vi "Begin.vi"(8 "error in":errorcluster) -> (0 "error out":errorcluster)   [LabVIEW 2018]
doc: "Called before other user functions, this VI is expected to open initial I/O refnums, load in file data, and do all program initialization. Notice that the <B>error out</B> terminal is simply used for data flow. Wiring it to other structures or subVIs ensures that this VI runs first."
uses:
  <vilib>/Rock Robotics/WPI/DriverStation/WPI_DriverStationRobotMode2.ctl
  Typedefs/typedef_enum_Begin_State.ctl
  <vilib>/Rock Robotics/WPI/Joystick/WPI_JoystickDeviceEnum.ctl
  Typedefs/typedef_enum_refnums.ctl
  <vilib>/Rock Robotics/WPI/SafetyOutput/WPI_SafetyOutputConfigMenu.ctl
  <vilib>/Rock Robotics/SystemInterfaces/DIO/FPGA_DIOChannel.ctl
  <vilib>/Rock Robotics/SystemInterfaces/DIO/FPGA_DIOPWMChannel.ctl
  <vilib>/Rock Robotics/WPI/Solenoid/WPI_SolenoidChannel.ctl
  <vilib>/Rock Robotics/WPI/ThirdParty/Phoenix-LabVIEW/Motor Controller/Controls/CTRE_Phoenix_MotorControl_FeedbackDevice.ctl
  Robot Global Data.vi
  <vilib>/Rock Robotics/Network Tables/NT Write Number.vi
  <vilib>/Rock Robotics/WPI/Counter/WPI_CounterDigitalInputToDigitalSource.vi
  <vilib>/Rock Robotics/WPI/RobotDrive/WPI_RobotDriveOpen4MotorWithSPARK.vi
  <vilib>/Rock Robotics/WPI/MotorControl/WPI_MotorControlOpen SPARK.vi
  <vilib>/Rock Robotics/WPI/Switch/WPI_SwitchOpenLimit.vi
  <vilib>/Rock Robotics/WPI/Solenoid/WPI_SolenoidOpenDouble.vi
  <vilib>/Rock Robotics/WPI/Utilities/WPI_GetSetVariantRefNum.vi
  <vilib>/Rock Robotics/Network Tables/NT Write String Array.vi
  <vilib>/Rock Robotics/WPI/Gyro/WPI_GyroXRS450_SPI_Open.vi
  <vilib>/Rock Robotics/SystemInterfaces/spilib/spi_bus.ctl
  <vilib>/Rock Robotics/SystemInterfaces/AI/FPGA_AIChannel.ctl
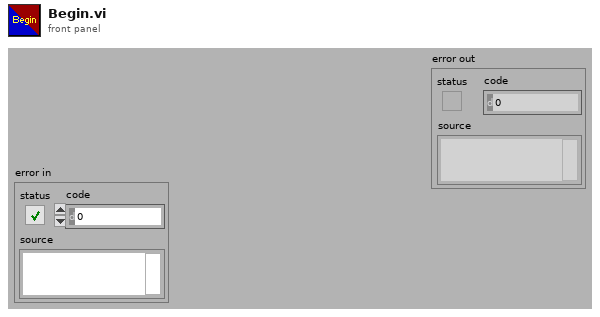
[diagram p1: front panel]
types:
  T1 = typedef "typedef_enum_Begin_State.ctl" = enum16{"Network_Setup", "Joy_Stick_Setup", "Drive_Train_Setup", "Ball_Intake_Setup", "Wrist_Setup", "Hatch_Deploy_Setup", "Compressor_Setup", "Lift_Setup", "Gyro_Setup", "Stop"}
  T2 = typedef "WPI_DriverStationRobotMode2.ctl" = enum16{"Autonomous Disabled", "Autonomous Enabled", "Teleop Disabled", "Teleop Enabled", "Disconnected", "Finish", "Test Disabled", "Test Enabled", "Emergency Stopped"}
  T3 = typedef "typedef_enum_refnums.ctl" = enum16{"Joy_L", "Joy_R", "Drive_Motors", "Intake_Motor", "Wrist_Solenoid", "Hatch_Solenoid", "Compressor", "Lift_Motor", "Lift_Motor_2", "Gyro", "Drive_Enc_L", "Drive_Enc_R", "Lift_Lower_Limit", "Lift_Upper_Limit", "Ball_Switch", "Jump_Solenoid"}
  T4 = typedef "WPI_JoystickDeviceEnum.ctl" = enum16{"USB 0", "USB 1", "USB 2", "USB 3", "USB 4", "USB 5"}
  T5 = typedef "WPI_SafetyOutputConfigMenu.ctl" = enum16{"Enable", "Disable"}
  T6 = typedef "FPGA_DIOPWMChannel.ctl" = enum8{"PWM 0", "PWM 1", "PWM 2", "PWM 3", "PWM 4", "PWM 5", "PWM 6", "PWM 7", "PWM 8", "PWM 9", "PWM MXP 0", "PWM MXP 1", "PWM MXP 2", "PWM MXP 3", "PWM MXP 4", "PWM MXP 5", "PWM MXP 6", "PWM MXP 7", "PWM MXP 8", "PWM MXP 9", "Invalid"}
  T7 = typedef "WPI_SolenoidChannel.ctl" = enum8{"Solenoid 0", "Solenoid 1", "Solenoid 2", "Solenoid 3", "Solenoid 4", "Solenoid 5", "Solenoid 6", "Solenoid 7", "Invalid"}
  T8 = typedef "FPGA_DIOChannel.ctl" = enum8{"DIO 0", "DIO 1", "DIO 2", "DIO 3", "DIO 4", "DIO 5", "DIO 6", "DIO 7", "DIO 8", "DIO 9", "DIO MXP 0", "DIO MXP 1", "DIO MXP 2", "DIO MXP 3", "DIO MXP 4", "DIO MXP 5", "DIO MXP 6", "DIO MXP 7", "DIO MXP 8", "DIO MXP 9", "DIO MXP 10", "DIO MXP 11", "DIO MXP 12", "DIO MXP 13", "DIO MXP 14", "DIO MXP 15", "SPI Port CS1", "SPI Port CS2", "SPI Port CS3", "SPI Port MISO", "SPI Port MOSI", "Invalid"}
  T9 = enum16{"FollowerType_PercentOutput", "FollowerType_AuxOutput1"}
  T10 = typedef "spi_bus.ctl" = enum16{"SPI On-Board, CS0", "SPI On-Board, CS1", "SPI On-Board, CS2", "SPI On-Board, CS3", "SPI MXP", "Invalid"}
  T11 = typedef "typedef_enum_refnums.ctl" = enum16{"Joy_L", "Joy_R", "Drive_Motors", "Intake_Motor", "Wrist_Solenoid", "Hatch_Solenoid", "Compressor", "Lift_Motor", "Lift_Motor_2", "Gyro", "Potentio", "Drive_Enc_L", "Drive_Enc_R", "Lift_Lower_Limit", "Lift_Upper_Limit", "Ball_Switch", "Jump_Solenoid"}
  T12 = typedef "FPGA_AIChannel.ctl" = enum8{"AI 0", "AI 1", "AI 2", "AI 3", "AI MXP 0", "AI MXP 1", "AI MXP 2", "AI MXP 3", "Invalid"}
  T13 = typedef "WPI_JoystickDevRef.ctl" = cluster{"Device":T4}
  T14 = typedef "WPI_RobotDriveDevRef.ctl" = cluster{"DevStatus":errorcluster, "Motors[]":T15[], "Square Inputs":bool, "Max Output":dbl}
  T15 = typedef "WPI_MotorControlDeviceRef.ctl" = cluster{"DeviceStatus":errorcluster, "Type":T16, "PWM":cluster{"PWM Channel":T6, "DeadBand":T17}, "CAN":cluster{"Device Number":u8, "SetOutput VI Ref":variant, "GetOutput VI Ref":variant, "Enable VI Ref":variant, "Disable VI Ref":variant, "Data":variant}, "Invert":bool, "DIO PWM":cluster{"PWM \"Enable\" Channel":T6, "DIOChannel":T8, "PWM Rate":dbl}}
  T16 = typedef "WPI_MotorControlType.ctl" = enum16{"PWM", "CAN", "DIO PWM"}
  T17 = typedef "WPI_PWMDeadband.ctl" = cluster{"Name":string, "maxPositivePwm":i32, "minPositivePwm":i32, "centerPwm":i32, "maxNegativePwm":i32, "minNegativePwm":i32, "angularRange":u16}
  T18 = typedef "WPI_DigitalInputDevRef.ctl" = cluster{"DevStatus":errorcluster, "DIO Channel":T8}
  T19 = typedef "FPGA_CounterEncoderSourceConvertionLVSourceType.ctl" = cluster{"DevStatus":errorcluster, "AnalogTriggerMode?":bool, "DigitalMode":cluster{"DIO Channel":T20}, "AnalogTriggerMode":cluster{"AnalogTriggerIndex":T21, "OutputType":T22}}
  T20 = typedef "FPGA_DIODigitalSourceChannel.ctl" = enum8{"DIO 0", "DIO 1", "DIO 2", "DIO 3", "DIO 4", "DIO 5", "DIO 6", "DIO 7", "DIO 8", "DIO 9", "DIO MXP 0", "DIO MXP 1", "DIO MXP 2", "DIO MXP 3", "DIO MXP 4", "DIO MXP 5", "DIO MXP 6", "DIO MXP 7", "DIO MXP 8", "DIO MXP 9", "DIO MXP 10", "DIO MXP 11", "DIO MXP 12", "DIO MXP 13", "DIO MXP 14", "DIO MXP 15", "SPI Port CS1", "SPI Port CS2", "SPI Port CS3", "SPI Port MISO", "SPI Port MOSI", "Disabled"}
  T21 = typedef "FPGA_AnalogTriggerIndex.ctl" = enum8{"Trig 0", "Trig 1", "Trig 2", "Trig 3", "Trig 4", "Trig 5", "Trig 6", "Trig 7", "Invalid"}
  T22 = typedef "FPGA_AnalogTriggerOutType.ctl" = enum16{"InWindow", "TriggerState", "Rising", "Falling"}
  T23 = typedef "WPI_EncoderDevRef.ctl" = cluster{"DevStatus":errorcluster, "EncoderIndex":T24, "CounterIndex":T25, "DistancePerCount":dbl, "Decoding Type":T26}
  T24 = typedef "FPGA_EncoderIdx.ctl" = enum8{"Enc 0", "Enc 1", "Enc 2", "Enc 3", "Enc 4", "Enc 5", "Enc 6", "Enc 7", "Invalid"}
  T25 = typedef "FPGA_CounterCtrSystemIndex.ctl" = enum8{"Ctr 0", "Ctr 1", "Ctr 2", "Ctr 3", "Ctr 4", "Ctr 5", "Ctr 6", "Ctr 7", "Invalid"}
  T26 = typedef "WPI_EncoderType.ctl" = enum16{"1x", "2x", "4x"}
  T27 = typedef "WPI_SwitchDevRef.ctl" = cluster{"DevStatus":errorcluster, "DIO Channel":T8, "CntIndex":T25, "Normally Closed":bool}
  T28 = typedef "WPI_SolenoidDevRef.ctl" = cluster{"DevStatus":errorcluster, "Pneumatics Control Module":u8, "Forward Solenoid Channel":T7, "Reverse Solenoid Channel":T7}
  T29 = typedef "WPI_CompressorDevRef.ctl" = cluster{"DevStatus":errorcluster, "Pneumatics Control Module":u8}
  T30 = typedef "CTRE_Phoenix_MotorControl_FeedbackDevice.ctl" = i8
  T31 = typedef "WPI_GyroDevRef.ctl" = cluster{"DevStatus":errorcluster, "Analog Channel":T12, "Gain (VoltsPerDegree/Second)":dbl, "Gyro Type":enum16{"Analog", "XRS450"}, "Handle":i32, "SPI Bus":T10, "Device Found":bool, "Sample Rate":dbl, "Calibrate On Open":bool, "Offset":dbl}
  T32 = typedef "WPI_PotentiometerDevRef.ctl" = cluster{"DevStatus":errorcluster, "Analog Channel":T12, "Invert Output":bool}
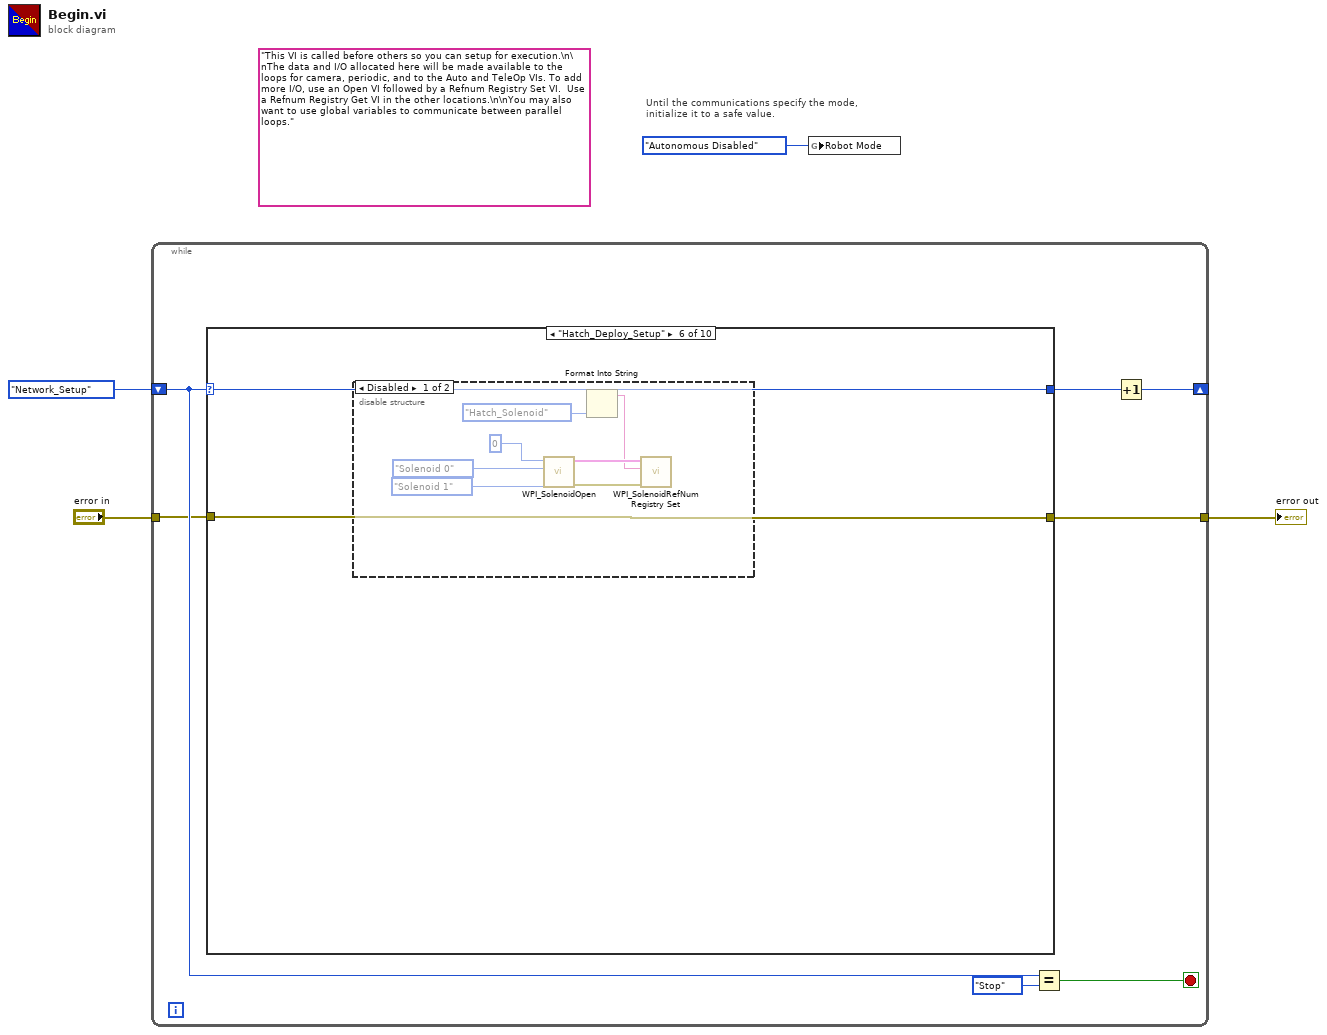
[diagram p0: block diagram]
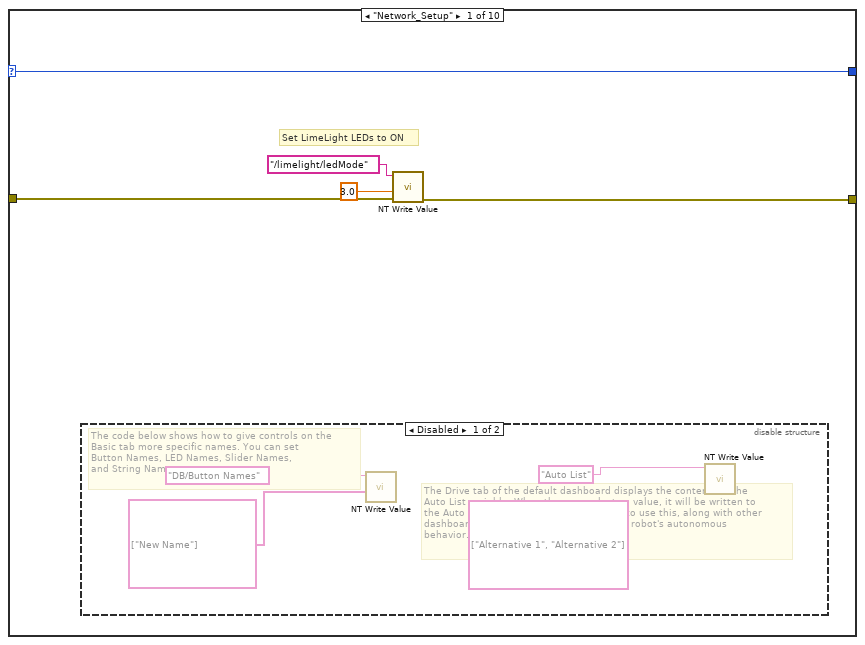
[diagram p2: hidden frame]
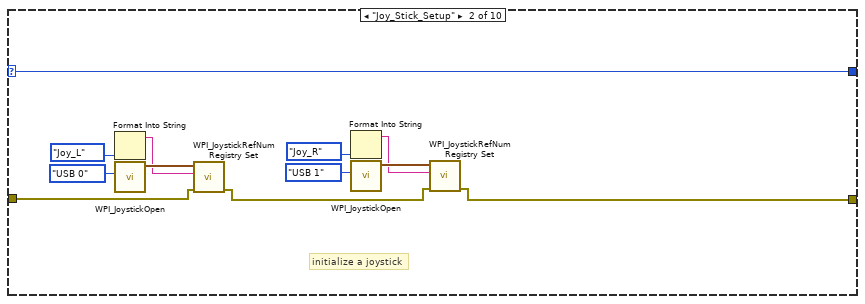
[diagram p4: hidden frame]
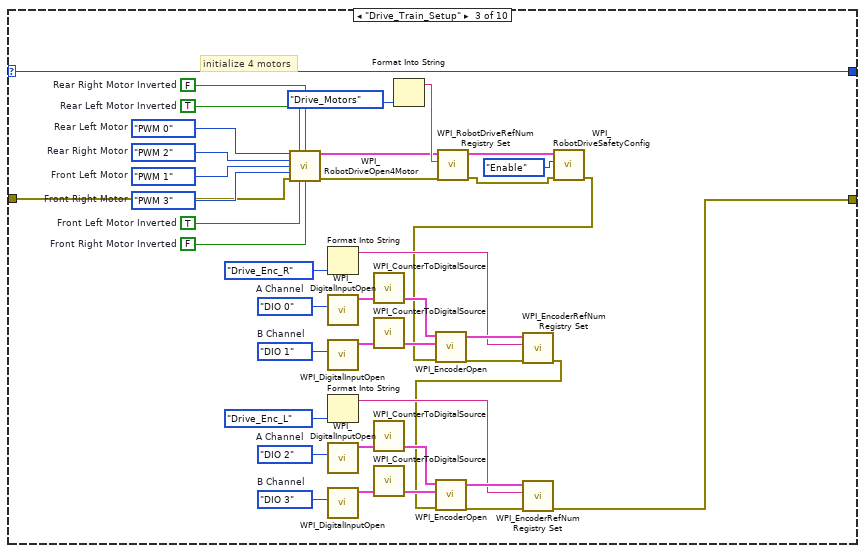
[diagram p5: hidden frame]
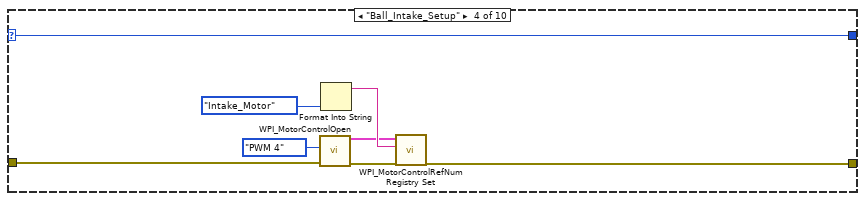
[diagram p6: hidden frame]
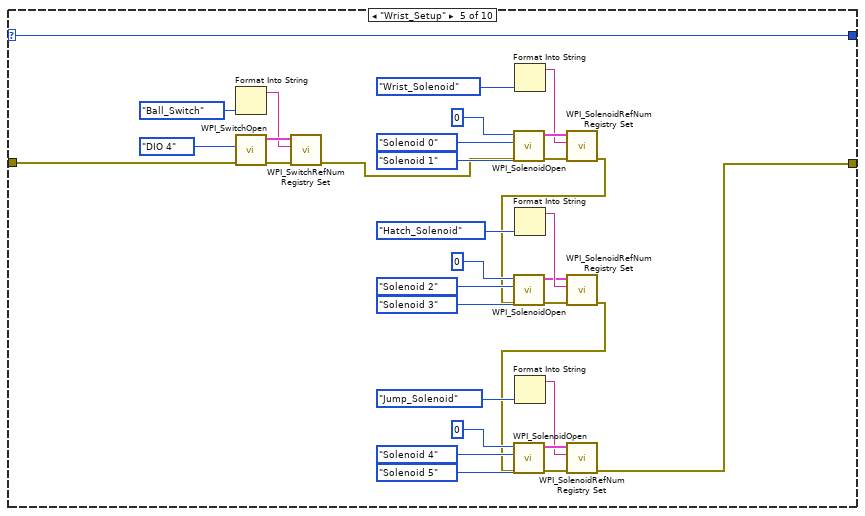
[diagram p7: hidden frame]
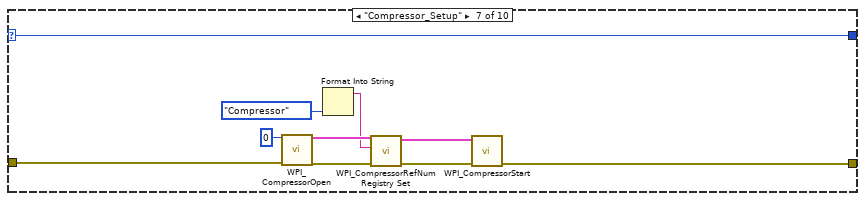
[diagram p9: hidden frame]
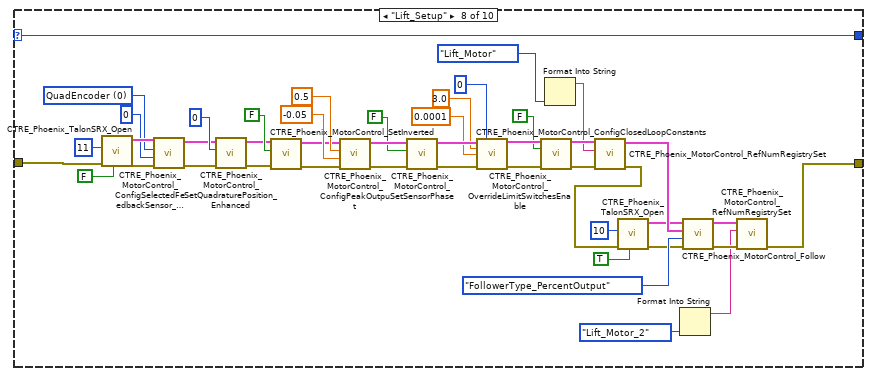
[diagram p10: hidden frame]
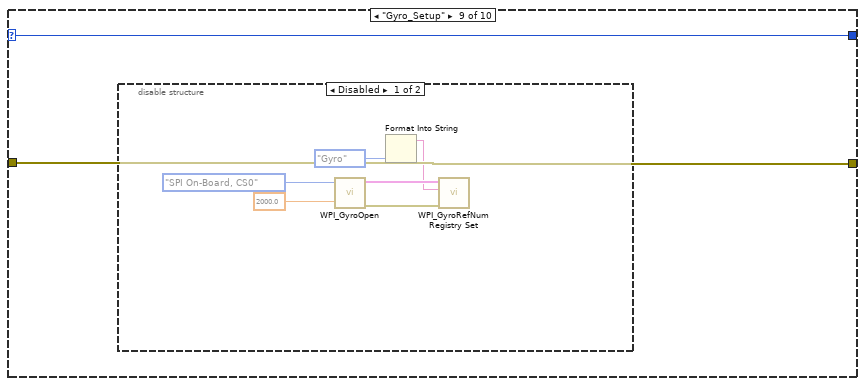
[diagram p11: hidden frame]
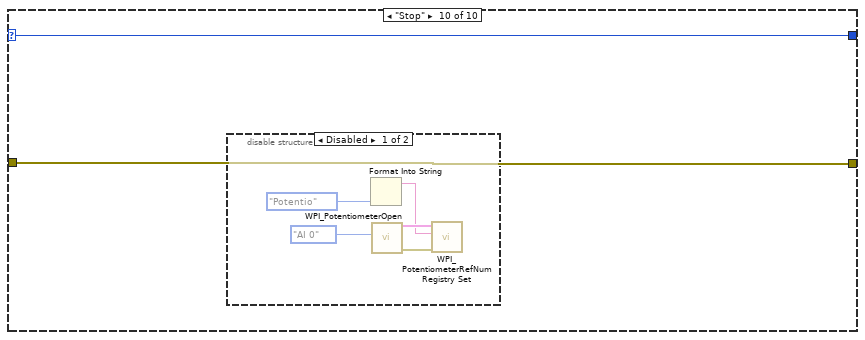
[diagram p13: hidden frame]
diagram:
  (unwired) "This VI is called before others so you can setup for execution.\n\nThe data and I/O allocated here will be made available to the loops for camera, periodic, and to the Auto and TeleOp VIs. To add more I/O, use an Open VI followed by a Refnum Registry Set VI.  Use a Refnum Registry Get VI in the other locations.\n\nYou may also want to use global variables to communicate between parallel loops."
  # "Until the communications specify the mode,\ninitialize it to a safe value."
  n1 = while {
    shift-right: [w10] -> _
    shift-left: typedef_enum_Begin_State."Network_Setup" ("Enum") -> [w8]
    tunnel: "error in" -> [w6]
    tunnel: [w5] -> w1
    stop <- w9 stop-if-true
    n2 = case shown="\"Hatch_Deploy_Setup\"" w8 {
      selector: w8 -> [w16 w32 w72 w80 w112 w114 w131 w176 w178 w186]
      tunnel: [w16 w32 w72 w80 w112 w114 w131 w176 w178 w186] -> w11
      tunnel: w6 -> [w13 w23 w38 w74 w85 w113 w123 w140 w177 w185]
      tunnel: [w12 w22 w33 w73 w81 w113 w122 w132 w177 w185] -> w5
      frame "Network_Setup" {
        # "Set LimeLight LEDs to ON"
        n3 = disable-structure shown="Disabled" {
          frame Disabled {
            # "The Drive tab of the default dashboard displays the contents of the\nAuto List variable. When the user selects a value, it will be written to\nthe Auto Selector variable. You may want to use this, along with other\ndashboard inputs, to let drivers define the robot's autonomous\nbehavior."
            # "The code below shows how to give controls on the\nBasic tab more specific names. You can set\nButton Names, LED Names, Slider Names,\nand String Names."
            n4 = call-poly <vilib>:"NT Write Value.vi"("String Array"=string[] ["New Name"], "Name"="DB/Button Names") -> ()  [unwired: 9 in, 1 out]
            n5 = call-poly <vilib>:"NT Write Value.vi"("String Array"=string[] ["Alternative 1", "Alternative 2"], "Name"="Auto List") -> ()  [unwired: 9 in, 1 out]
          }
          frame Enabled {
          }
        }
        n6 = call-poly <vilib>:"NT Write Value.vi"("error in"=w13, "Numeric"=3.0, "Name"="/limelight/ledMode") -> ("error out"=w12:errorcluster)  [unwired: 8 in]
      }
      frame "Joy_Stick_Setup" {
        # "initialize a joystick"
        n7 = Format Into String(typedef_enum_refnums."Joy_L" ("Enum")) -> (resulting string=w26:string)  [unwired: 3 in, 1 out]
        n8 = call <vilib>:"WPI_JoystickOpen.vi"("JoystickDevice"=WPI_JoystickDeviceEnum."USB 0") -> ("JoystickDevRef"=w28:T13)  [unwired: 10 in]
        n9 = call <vilib>:"WPI_JoystickRefNum Registry Set.vi"("error in (no error)"=w23, "refnum name"=w26, "JoystickDevRef"=w28) -> ("error out"=w21:errorcluster)  [unwired: 7 in, 1 out]
        n10 = Format Into String(typedef_enum_refnums."Joy_R" ("Enum")) -> (resulting string=w24:string)  [unwired: 3 in, 1 out]
        n11 = call <vilib>:"WPI_JoystickOpen.vi"("JoystickDevice"=WPI_JoystickDeviceEnum."USB 1") -> ("JoystickDevRef"=w31:T13)  [unwired: 10 in]
        n12 = call <vilib>:"WPI_JoystickRefNum Registry Set.vi"("error in (no error)"=w21, "refnum name"=w24, "JoystickDevRef"=w31) -> ("error out"=w22:errorcluster)  [unwired: 7 in, 1 out]
      }
      frame "Drive_Train_Setup" {
        w39 = FALSE  # Rear Right Motor Inverted
        w40 = TRUE  # Front Left Motor Inverted
        w41 = FALSE  # Front Right Motor Inverted
        w42 = TRUE  # Rear Left Motor Inverted
        w43 = FPGA_DIOPWMChannel."PWM 3"  # Front Right Motor
        w44 = FPGA_DIOPWMChannel."PWM 1"  # Front Left Motor
        w45 = FPGA_DIOPWMChannel."PWM 2"  # Rear Right Motor
        w46 = FPGA_DIOPWMChannel."PWM 0"  # Rear Left Motor
        w57 = FPGA_DIOChannel."DIO 3"  # B Channel
        w56 = FPGA_DIOChannel."DIO 2"  # A Channel
        w67 = FPGA_DIOChannel."DIO 1"  # B Channel
        w66 = FPGA_DIOChannel."DIO 0"  # A Channel
        # "initialize 4 motors"
        n13 = call-poly <vilib>:"WPI_RobotDriveOpen4Motor.vi"("Rear Left Motor"=w46, "Rear Left Motor Inverted"=w42, "Rear Right Motor Inverted"=w39, "Rear Right Motor"=w45, "Front Left Motor"=w44, "Front Right Motor"=w43, "error in (no error)"=w38, "Front Left Motor Inverted"=w40, "Front Right Motor Inverted"=w41) -> ("RobotDriveDevRef"=w47:T14, "error out"=w37:errorcluster)  [unwired: 5 in]
        n14 = Format Into String(typedef_enum_refnums."Drive_Enc_R" ("Enum")) -> (resulting string=w59:string)  [unwired: 3 in, 1 out]
        n15 = call <vilib>:"WPI_DigitalInputOpen.vi"("DIO Channel"=w66) -> ("DigitalInputDevRef"=w63:T18)  [unwired: 1 in, 9 out]
        n16 = call <vilib>:"WPI_DigitalInputOpen.vi"("DIO Channel"=w67) -> ("DigitalInputDevRef"=w64:T18)  [unwired: 1 in, 9 out]
        n17 = Format Into String(typedef_enum_refnums."Drive_Enc_L" ("Enum")) -> (resulting string=w49:string)  [unwired: 3 in, 1 out]
        n18 = call <vilib>:"WPI_DigitalInputOpen.vi"("DIO Channel"=w56) -> ("DigitalInputDevRef"=w53:T18)  [unwired: 1 in, 9 out]
        n19 = call <vilib>:"WPI_DigitalInputOpen.vi"("DIO Channel"=w57) -> ("DigitalInputDevRef"=w54:T18)  [unwired: 1 in, 9 out]
        n20 = call-poly <vilib>:"WPI_CounterToDigitalSource.vi"("DigitalInputDevRef"=w63) -> ("Digital Source"=w62:T19)  [unwired: 6 out]
        n21 = call-poly <vilib>:"WPI_CounterToDigitalSource.vi"("DigitalInputDevRef"=w64) -> ("Digital Source"=w65:T19)  [unwired: 6 out]
        n22 = call-poly <vilib>:"WPI_CounterToDigitalSource.vi"("DigitalInputDevRef"=w53) -> ("Digital Source"=w52:T19)  [unwired: 6 out]
        n23 = call-poly <vilib>:"WPI_CounterToDigitalSource.vi"("DigitalInputDevRef"=w54) -> ("Digital Source"=w55:T19)  [unwired: 6 out]
        n24 = Format Into String(typedef_enum_refnums."Drive_Motors" ("Enum")) -> (resulting string=w68:string)  [unwired: 3 in, 1 out]
        n25 = call <vilib>:"WPI_RobotDriveRefNum Registry Set.vi"("error in (no error)"=w37, "refnum name"=w68, "RobotDriveDevRef"=w47) -> ("error out"=w36:errorcluster, "RobotDriveDevRef"=w71:T14)  [unwired: 1 in, 6 out]
        n26 = call <vilib>:"WPI_RobotDriveSafetyConfig.vi"("error in (no error)"=w36, "mode"=WPI_SafetyOutputConfigMenu."Enable", "RobotDriveDevRef"=w71) -> ("error out"=w35:errorcluster)  [unwired: 7 in, 1 out]
        n27 = call <vilib>:"WPI_EncoderOpen.vi"("error in (no error)"=w35, "BSource"=w65, "ASource"=w62) -> ("error out"=w60:errorcluster, "EncoderDevRef"=w61:T23)  [unwired: 5 in, 2 out]
        n28 = call <vilib>:"WPI_EncoderRefNum Registry Set.vi"("error in (no error)"=w60, "refnum name"=w59, "EncoderDevRef"=w61) -> ("error out"=w34:errorcluster)  [unwired: 7 in, 1 out]
        n29 = call <vilib>:"WPI_EncoderOpen.vi"("error in (no error)"=w34, "BSource"=w55, "ASource"=w52) -> ("error out"=w50:errorcluster, "EncoderDevRef"=w51:T23)  [unwired: 5 in, 2 out]
        n30 = call <vilib>:"WPI_EncoderRefNum Registry Set.vi"("error in (no error)"=w50, "refnum name"=w49, "EncoderDevRef"=w51) -> ("error out"=w33:errorcluster)  [unwired: 7 in, 1 out]
      }
      frame "Ball_Intake_Setup" {
        n31 = call-poly <vilib>:"WPI_MotorControlOpen.vi"("error in (no error)"=w74, "PWM Channel"=FPGA_DIOPWMChannel."PWM 4") -> ("error out"=w76:errorcluster, "MotorControlDeviceRef"=w75:T15)  [unwired: 8 in]
        n32 = Format Into String(typedef_enum_refnums."Intake_Motor" ("Enum")) -> (resulting string=w77:string)  [unwired: 3 in, 1 out]
        n33 = call <vilib>:"WPI_MotorControlRefNum Registry Set.vi"("error in (no error)"=w76, "refnum name"=w77, "MotorControlDevRef"=w75) -> ("error out"=w73:errorcluster)  [unwired: 7 in, 1 out]
      }
      frame "Wrist_Setup" {
        n34 = Format Into String(typedef_enum_refnums."Ball_Switch" ("Enum")) -> (resulting string=w100:string)  [unwired: 3 in, 1 out]
        n35 = call-poly <vilib>:"WPI_SwitchOpen.vi"("error in (no error)"=w85, "DIO Channel"=FPGA_DIOChannel."DIO 4") -> ("error out"=w102:errorcluster, "SwitchDevRef"=w103:T27)  [unwired: 8 in]
        n36 = call <vilib>:"WPI_SwitchRefNum Registry Set.vi"("error in (no error)"=w102, "refnum name"=w100, "SwitchDevRef"=w103) -> ("error out"=w84:errorcluster)  [unwired: 7 in, 1 out]
        n37 = call-poly <vilib>:"WPI_SolenoidOpen.vi"("error in (no error)"=w84, "Reverse Solenoid Channel"=WPI_SolenoidChannel."Solenoid 1", "Forward Solenoid Channel"=WPI_SolenoidChannel."Solenoid 0", "Pneumatics Control Module (0)"=u8 0) -> ("error out"=w110:errorcluster, "SolenoidDevRef"=w111:T28)  [unwired: 6 in]
        n38 = Format Into String(typedef_enum_refnums."Wrist_Solenoid" ("Enum")) -> (resulting string=w105:string)  [unwired: 3 in, 1 out]
        n39 = Format Into String(typedef_enum_refnums."Hatch_Solenoid" ("Enum")) -> (resulting string=w99:string)  [unwired: 3 in, 1 out]
        n40 = Format Into String(typedef_enum_refnums."Jump_Solenoid" ("Enum")) -> (resulting string=w86:string)  [unwired: 3 in, 1 out]
        n41 = call <vilib>:"WPI_SolenoidRefNum Registry Set.vi"("error in (no error)"=w110, "refnum name"=w105, "SolenoidDevRef"=w111) -> ("error out"=w83:errorcluster)  [unwired: 7 in, 1 out]
        n42 = call-poly <vilib>:"WPI_SolenoidOpen.vi"("error in (no error)"=w83, "Reverse Solenoid Channel"=WPI_SolenoidChannel."Solenoid 3", "Forward Solenoid Channel"=WPI_SolenoidChannel."Solenoid 2", "Pneumatics Control Module (0)"=u8 0) -> ("error out"=w94:errorcluster, "SolenoidDevRef"=w93:T28)  [unwired: 6 in]
        n43 = call <vilib>:"WPI_SolenoidRefNum Registry Set.vi"("error in (no error)"=w94, "refnum name"=w99, "SolenoidDevRef"=w93) -> ("error out"=w82:errorcluster)  [unwired: 7 in, 1 out]
        n44 = call-poly <vilib>:"WPI_SolenoidOpen.vi"("error in (no error)"=w82, "Reverse Solenoid Channel"=WPI_SolenoidChannel."Solenoid 5", "Forward Solenoid Channel"=WPI_SolenoidChannel."Solenoid 4", "Pneumatics Control Module (0)"=u8 0) -> ("error out"=w91:errorcluster, "SolenoidDevRef"=w92:T28)  [unwired: 6 in]
        n45 = call <vilib>:"WPI_SolenoidRefNum Registry Set.vi"("error in (no error)"=w91, "refnum name"=w86, "SolenoidDevRef"=w92) -> ("error out"=w81:errorcluster)  [unwired: 7 in, 1 out]
      }
      frame "Hatch_Deploy_Setup" {
        n46 = disable-structure shown="Disabled" {
          frame Disabled {
            n47 = call-poly <vilib>:"WPI_SolenoidOpen.vi"("Reverse Solenoid Channel"=WPI_SolenoidChannel."Solenoid 1", "Forward Solenoid Channel"=WPI_SolenoidChannel."Solenoid 0", "Pneumatics Control Module (0)"=u8 0) -> ("error out"=w120:errorcluster, "SolenoidDevRef"=w121:T28)  [unwired: 7 in]
            n48 = Format Into String(typedef_enum_refnums."Hatch_Solenoid" ("Enum")) -> (resulting string=w115:string)  [unwired: 3 in, 1 out]
            n49 = call <vilib>:"WPI_SolenoidRefNum Registry Set.vi"("error in (no error)"=w120, "refnum name"=w115, "SolenoidDevRef"=w121) -> ()  [unwired: 7 in, 2 out]
          }
          frame Enabled {
          }
        }
      }
      frame "Compressor_Setup" {
        n50 = call <vilib>:"WPI_CompressorOpen.vi"("Pneumatics Control Module (0)"=u8 0, "error in (no error)"=w123) -> ("CompressorDevRef"=w130:T29, "error out"=w129:errorcluster)  [unwired: 12 in]
        n51 = Format Into String(typedef_enum_refnums."Compressor" ("Enum")) -> (resulting string=w126:string)  [unwired: 3 in, 1 out]
        n52 = call <vilib>:"WPI_CompressorRefNum Registry Set.vi"("error in (no error)"=w129, "refnum name"=w126, "CompressorDevRef"=w130) -> ("error out"=w125:errorcluster, "CompressorDevRef"=w124:T29)  [unwired: 7 in]
        n53 = call <vilib>:"WPI_CompressorStart.vi"("error in (no error)"=w125, "CompressorDevRef"=w124) -> ("error out"=w122:errorcluster)  [unwired: 8 in, 1 out]
      }
      frame "Lift_Setup" {
        w172 = T30 0 items=["QuadEncoder"=0, "Analog"=2, "Tachometer"=4, "Pulse Width Encoded Position"=8, "Sensor Sum (S0 + S1)"=9, "Sensor Difference (D0 - D1)"=10, "Remote Source 0"=11, "Remote Source 1"=12, "Software Emulated"=15] ("Feedback Device")
        n54 = call <vilib>:"CTRE_Phoenix_TalonSRX_Open.vi"("Invert"=FALSE, "error in"=w140, "Device Number"=u8 11) -> ("error out"=w173:errorcluster, "CAN Talon SRX Ref"=w174:T15)  [unwired: 7 in]
        n55 = call <vilib>:"CTRE_Phoenix_MotorControl_ConfigSelectedFeedbackSensor_Enhanced.vi"("error in (no error)"=w173, "pidLoopIdx"=0, "Feedback Device"=w172, "PhoenixMotorControlDevRef"=w174) -> ("error out"=w160:errorcluster, "PhoenixMotorControlDevRef"=w158:T15)  [unwired: 6 in]
        n56 = call <vilib>:"CTRE_Phoenix_MotorControl_SetQuadraturePosition_Enhanced.vi"("error in (no error)"=w160, "New Position"=0, "PhoenixMotorControlDevRef"=w158) -> ("error out"=w162:errorcluster, "PhoenixMotorControlDevRef"=w161:T15)  [unwired: 7 in]
        n57 = call <vilib>:"CTRE_Phoenix_MotorControl_SetInverted.vi"("error in (no error)"=w162, "Invert?"=FALSE, "PhoenixMotorControlDevRef"=w161) -> ("error out"=w168:errorcluster, "PhoenixMotorControlDevRef"=w167:T15)  [unwired: 7 in]
        n58 = call <vilib>:"CTRE_Phoenix_MotorControl_ConfigPeakOutput.vi"("error in (no error)"=w168, "Reverse Peak Percent Output"=-0.05, "Forward Peak Percent Output"=0.5, "PhoenixMotorControlDevRef"=w167) -> ("error out"=w164:errorcluster, "PhoenixMotorControlDevRef"=w165:T15)  [unwired: 6 in]
        n59 = call <vilib>:"CTRE_Phoenix_MotorControl_SetSensorPhase.vi"("error in (no error)"=w164, "PhaseSensor"=FALSE, "PhoenixMotorControlDevRef"=w165) -> ("error out"=w150:errorcluster, "PhoenixMotorControlDevRef"=w151:T15)  [unwired: 7 in]
        n60 = call <vilib>:"CTRE_Phoenix_MotorControl_ConfigClosedLoopConstants.vi"("PhoenixMotorControlDevRef"=w151, "slotIdx"=0, "P"=3.0, "I"=0.0001, "error in (no error)"=w150) -> ("PhoenixMotorControlDevRef"=w146:T15, "error out"=w143:errorcluster)  [unwired: 9 in]
        n61 = call <vilib>:"CTRE_Phoenix_MotorControl_OverrideLimitSwitchesEnable.vi"("PhoenixMotorControlDevRef"=w146, "Override Limit Switch Enable?"=FALSE, "error in (no error)"=w143) -> ("PhoenixMotorControlDevRef"=w145:T15, "error out"=w144:errorcluster)  [unwired: 11 in]
        n62 = Format Into String(typedef_enum_refnums."Lift_Motor" ("Enum")) -> (resulting string=w138:string)  [unwired: 3 in, 1 out]
        n63 = call <vilib>:"CTRE_Phoenix_MotorControl_RefNumRegistrySet.vi"("error in (no error)"=w144, "refnum name"=w138, "PhoenixMotorControlDevRef"=w145) -> ("error out"=w133:errorcluster, "PhoenixMotorControlDevRef"=w155:T15)  [unwired: 7 in]
        n64 = call <vilib>:"CTRE_Phoenix_TalonSRX_Open.vi"("Invert"=TRUE, "error in"=w133, "Device Number"=u8 10) -> ("error out"=w153:errorcluster, "CAN Talon SRX Ref"=w154:T15)  [unwired: 7 in]
        n65 = Format Into String(typedef_enum_refnums."Lift_Motor_2" ("Enum")) -> (resulting string=w134:string)  [unwired: 3 in, 1 out]
        n66 = call <vilib>:"CTRE_Phoenix_MotorControl_Follow.vi"("error in (no error)"=w153, "FollowerType"=T9."FollowerType_PercentOutput", "Master Controller to Follow"=w155, "PhoenixMotorControlDevRef"=w154) -> ("error out"=w135:errorcluster, "PhoenixMotorControlDevRef"=w136:T15)  [unwired: 6 in]
        n67 = call <vilib>:"CTRE_Phoenix_MotorControl_RefNumRegistrySet.vi"("error in (no error)"=w135, "refnum name"=w134, "PhoenixMotorControlDevRef"=w136) -> ("error out"=w132:errorcluster)  [unwired: 7 in, 1 out]
      }
      frame "Gyro_Setup" {
        n68 = disable-structure shown="Disabled" {
          frame Disabled {
            n69 = call-poly <vilib>:"WPI_GyroOpen.vi"("Sample Rate (Hz)"=2000.0, "SPI Bus"=spi_bus."SPI On-Board, CS0") -> ("error out"=w181:errorcluster, "GyroDevRef"=w184:T31)  [unwired: 7 in, 1 out]
            n70 = Format Into String(typedef_enum_refnums."Gyro" ("Enum")) -> (resulting string=w180:string)  [unwired: 3 in, 1 out]
            n71 = call <vilib>:"WPI_GyroRefNum Registry Set.vi"("error in (no error)"=w181, "refnum name"=w180, "GyroDevRef"=w184) -> ()  [unwired: 7 in, 2 out]
          }
          frame Enabled {
          }
        }
      }
      frame "Stop" {
        n72 = disable-structure shown="Disabled" {
          frame Disabled {
            n73 = Format Into String(typedef_enum_refnums."Potentio" ("Enum")) -> (resulting string=w188:string)  [unwired: 3 in, 1 out]
            n74 = call <vilib>:"WPI_PotentiometerOpen.vi"("Analog Channel"=FPGA_AIChannel."AI 0") -> ("error out"=w190:errorcluster, "PotDevRef"=w191:T32)  [unwired: 9 in]
            n75 = call <vilib>:"WPI_PotentiometerRefNum Registry Set.vi"("error in (no error)"=w190, "refnum name"=w188, "PotDevRef"=w191) -> ()  [unwired: 7 in, 2 out]
          }
          frame Enabled {
          }
        }
      }
    }
    n76 = Equal?(x=w8, y=typedef_enum_Begin_State."Stop") -> (x = y?=w9:bool)
    n77 = Increment(x=w11) -> (x+1=w10:T1)
  }
  "error out" <- w1
  n78 = global write "Robot Global Data.vi" "Robot Mode"(WPI_DriverStationRobotMode2."Autonomous Disabled" ("Robot Mode")) -> ()
